vi "Read Config Dir.vi"(8 "error in (no error)":errorcluster, 11 "Camera Dir Dialog in":refnum<class "Camera Dir Dialog.lvclass">) -> (0 "error out":errorcluster, 2 "Config Dir":path=path "D:/Test XDisplay images", 3 "Camera Dir Dialog out":refnum<class "Camera Dir Dialog.lvclass">)   [LabVIEW 2014, in "Camera Dir Dialog.lvlib" / "Camera Dir Dialog.lvclass"]
uses:
  Camera Dir Dialog.lvclass
  Camera Dir Dialog.lvclass/Camera Dir Dialog.ctl
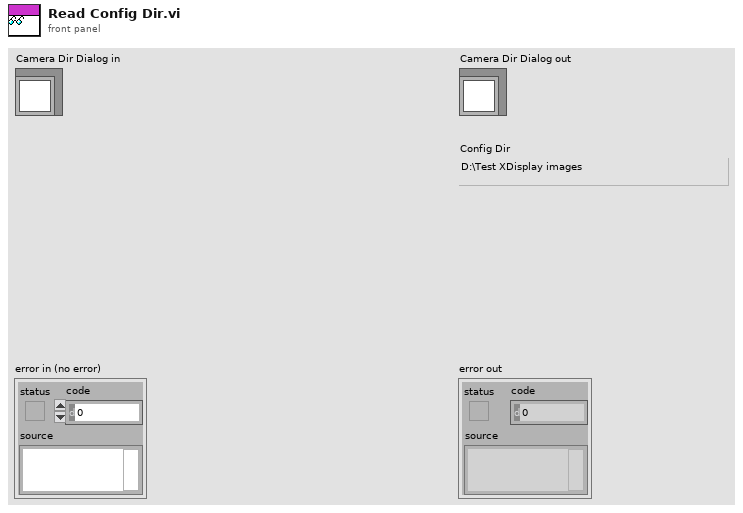
[diagram p1: front panel]
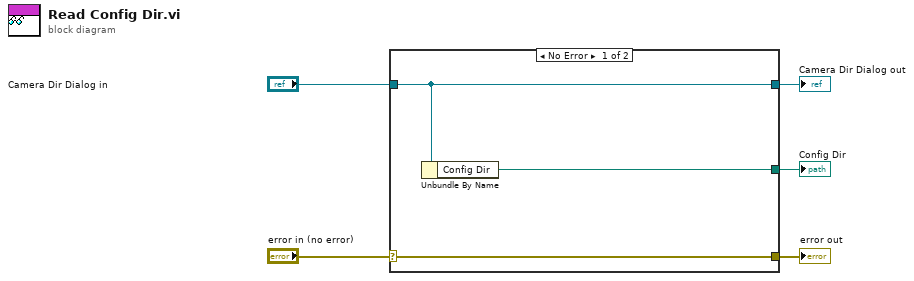
[diagram p0: block diagram]
diagram:
  n1 = case shown="No Error" "error in (no error)" {
    selector: "error in (no error)" -> [w8 w9]
    tunnel: [w8 w9] -> w4
    tunnel: [w7 w10] -> w2
    tunnel: "Camera Dir Dialog in" -> [w7 w10]
    tunnel: [w6 _] -> w1
    frame No Error {
      n2 = Unbundle By Name(w7) -> ("Config Dir"=w6:path)
    }
    frame Error {
    }
  }
  "error out" <- w4
  "Camera Dir Dialog out" <- w2
  "Config Dir" <- w1
